vi "Joystick 2 LiftSystem.vi"(11 "JoystickAxes":dbl[](array[numeric])) -> (3 "Lift Speed":dbl)   [LabVIEW 2018]
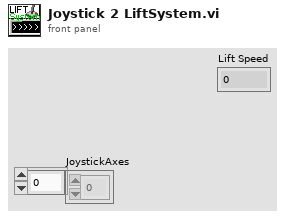
[diagram p1: front panel]
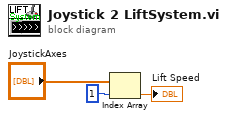
[diagram p0: block diagram]
diagram:
  n1 = Index Array(array="JoystickAxes", index=1) -> (element=→"Lift Speed":dbl)
